vi "Config DR.vi"(1 "DR":T1(ring)=enum."128SPS", 2 "Orig Config":u8[](array[numeric])) -> (0 "New Config":u8[](array[numeric]))   [LabVIEW 2021]
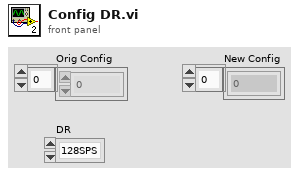
[diagram p1: front panel]
types:
  T1 = enum16{"8SPS", "16SPS", "32SPS", "64SPS", "128SPS", "250SPS", "475SPS", "860SPS"}
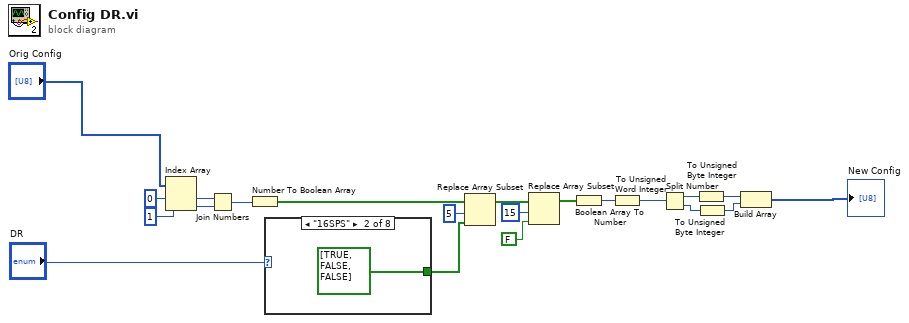
[diagram p0: block diagram]
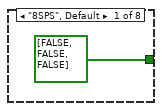
[diagram p2: hidden frame]
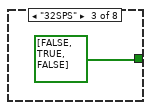
[diagram p3: hidden frame]
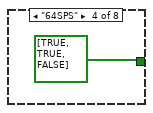
[diagram p4: hidden frame]
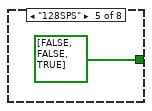
[diagram p5: hidden frame]
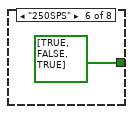
[diagram p6: hidden frame]
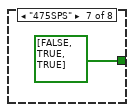
[diagram p7: hidden frame]
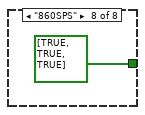
[diagram p8: hidden frame]
diagram:
  n1 = Index Array(array="Orig Config", index #1=0 ("index"), index #2=1 ("index")) -> (element #1=w4:u8, element #2=w5:u8)
  n2 = Join Numbers(hi=w4, lo=w5) -> ((hi.lo)=w6:u16)
  n3 = Number To Boolean Array(number=w6) -> (Boolean array=w7:bool[])
  n4 = case shown="\"16SPS\"" "DR" {
    tunnel: [bool[] [FALSE, FALSE, FALSE] bool[] [TRUE, FALSE, FALSE] bool[] [FALSE, TRUE, FALSE] bool[] [TRUE, TRUE, FALSE] bool[] [FALSE, FALSE, TRUE] bool[] [TRUE, FALSE, TRUE] bool[] [FALSE, TRUE, TRUE] bool[] [TRUE, TRUE, TRUE]] -> w9
    frame "8SPS", Default {
    }
    frame "16SPS" {
    }
    frame "32SPS" {
    }
    frame "64SPS" {
    }
    frame "128SPS" {
    }
    frame "250SPS" {
    }
    frame "475SPS" {
    }
    frame "860SPS" {
    }
  }
  n5 = Replace Array Subset(array=w7, new element=w9, index=5) -> (w17:bool[])
  n6 = Replace Array Subset(array=w17, new element=FALSE ("new element/subarray"), index=15) -> (w20:bool[])
  n7 = Boolean Array To Number(Boolean array=w20) -> (number=w14:u32)
  n8 = To Unsigned Word Integer(number=w14) -> (unsigned 16bit integer=w15:u16)
  n9 = Split Number(x=w15) -> (hi(x)=w10:u8, lo(x)=w12:u8)
  n10 = To Unsigned Byte Integer(number=w10) -> (unsigned 8bit integer=w11:u8)
  n11 = To Unsigned Byte Integer(number=w12) -> (unsigned 8bit integer=w13:u8)
  n12 = Build Array(w11, w13) -> (→"New Config":u8[])
